vi "max clamp working in light.vi"(0 "Image In":T4, 1 "Clamp Settings (Max Clamp 1)":T1={"Angle Range (+/-)"=10.0, "Edge Polarity"={"Start"=0, "End"=0}} {"Edge Polarity"."Start" items=["Any", "Rising", "Falling"]; "Edge Polarity"."End" items=["Any", "Rising", "Falling"]}, 7 "error in":errorcluster) -> (20 "Image Out":T4, 21 "Clamp Results (Max Clamp 1)":T3, 22 "Clamp Points (Max Clamp 1)":T2, 24 "X Average":dbl, 27 "error out":errorcluster)   [LabVIEW 2016]
uses:
  <vilib>/vision/Image Controls.llb/IMAQ Image.ctl
  <vilib>/vision/Pattern Matching.llb/IMAQ Curve Parameters.ctl
  <vilib>/vision/NI_Vision_Development_Module.lvlib
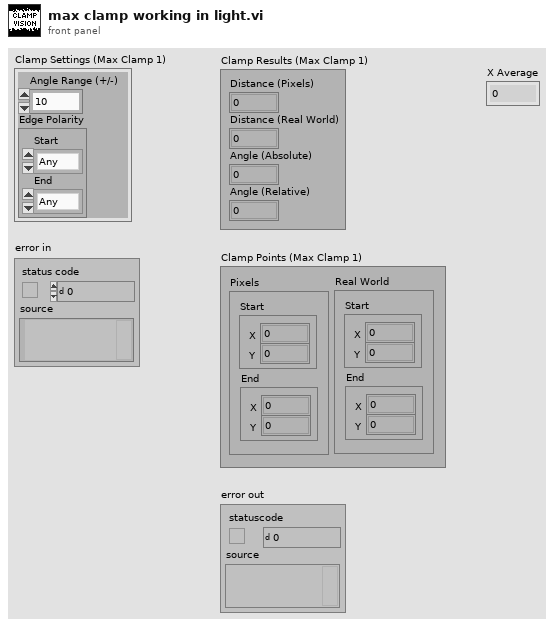
[diagram p1: front panel]
types:
  T1 = cluster{"Angle Range (+/-)":dbl, "Edge Polarity":cluster{"Start":u32, "End":u32}}
  T2 = cluster{"Pixels ":cluster{"Start":cluster{"X":dbl, "Y":dbl}, "End":cluster{"X":dbl, "Y":dbl}}, "Real World":cluster{"Start":cluster{"X":dbl, "Y":dbl}, "End":cluster{"X":dbl, "Y":dbl}}}
  T3 = cluster{"Distance (Pixels)":dbl, "Distance (Real World)":dbl, "Angle (Absolute)":dbl, "Angle (Relative)":dbl}
  T4 = typedef "IMAQ Image.ctl" = refnum<image>
  T5 = typedef "IMAQ Curve Parameters.ctl" = cluster{"Extraction Mode":u32, "Edge Threshold":i32, "Edge Filter Size":u32, "Min Length":i32, "Row Search Step Size":i32, "Col Search Step Size":i32, "Max Endpoint Gap":i32, "Closed":bool, "Subpixel":bool}
  T6 = cluster{"Show Search Area":bool, "Show Curves":bool, "Show Clamp Locations":bool, "Show Result":bool, "Search Area Color":u32, "Curves Color":u32, "Clamp Locations Color":u32, "Result Color":u32, "Overlay Group Name":string}
  T7 = cluster{"Global Rectangle":i32[], "Contours":cluster{"ID":enum32{"External", "Internal"}, "Type":u32, "Coordinates":i32[]}[]}
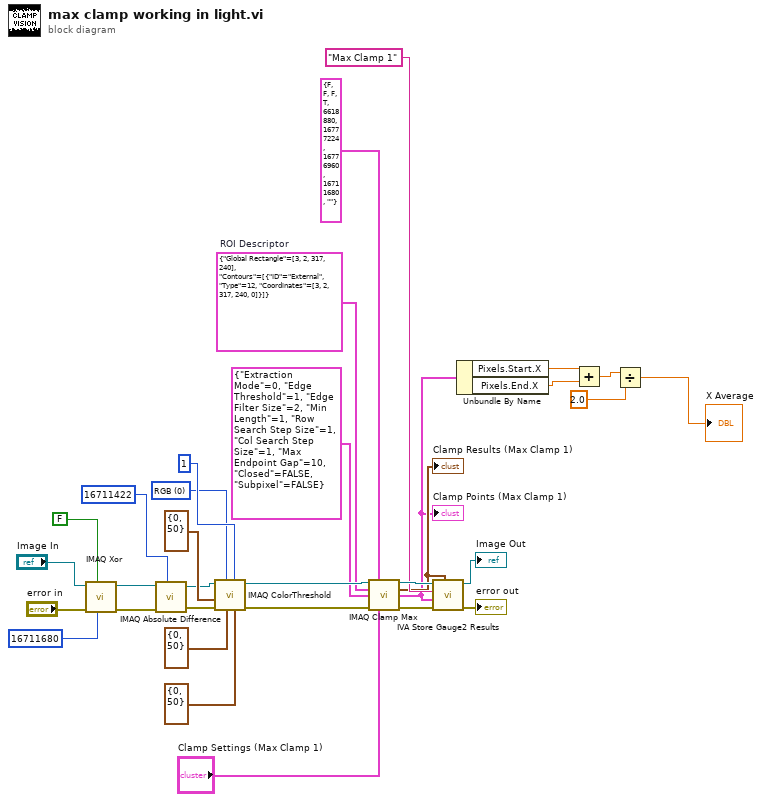
[diagram p0: block diagram]
diagram:
  w10 = T7 {"Global Rectangle"=[3, 2, 317, 240], "Contours"=[{"ID"=enum."External", "Type"=12, "Coordinates"=[3, 2, 317, 240, 0]}]}  # ROI Descriptor
  w24 = u16 0 items=["RGB", "HSL", "HSV", "HSI"] ("Color Mode")
  n1 = call "IMAQ Xor"("Constant"=16711680, "Xor/Xnor (Xor)"=FALSE, "error in (no error)"="error in", "Image Src A"="Image In") -> ("error out"=w27:errorcluster, "Image Dst Out"=w26:T4)  [unwired: 2 in, 4 out]
  n2 = call "IMAQ Absolute Difference"("Image Src A"=w26, "Constant"=16711422, "error in (no error)"=w27) -> ("Image Dst Out"=w20:T4, "error out"=w19:errorcluster)  [unwired: 2 in, 2 out]
  n3 = call "IMAQ ColorThreshold"("Blue or Luma or Val or Inten Range"=cluster{"Lower value":i32, "Upper value":i32} {"Lower value"=0, "Upper value"=50}, "Replace Value"=1, "Green or Sat Range"=cluster{"Lower value":i32, "Upper value":i32} {"Lower value"=0, "Upper value"=50}, "Color Mode"=w24, "error in (no error)"=w19, "Red or Hue Range"=cluster{"Lower value":i32, "Upper value":i32} {"Lower value"=0, "Upper value"=50}, "Image Src"=w20) -> ("error out"=w16:errorcluster, "Image Dst Out"=w17:T4)  [unwired: 1 in, 2 out]
  n4 = call "IMAQ Clamp Max"("Source Image"=w17, "Overlay Settings"=T6 {"Show Search Area"=FALSE, "Show Curves"=FALSE, "Show Clamp Locations"=FALSE, "Show Result"=TRUE, "Search Area Color"=6618880, "Curves Color"=16777224, "Clamp Locations Color"=16776960, "Result Color"=16711680, "Overlay Group Name"=""}, "ROI Descriptor"=w10, "Curve Extraction Settings"=T5 {"Extraction Mode"=0, "Edge Threshold"=1, "Edge Filter Size"=2, "Min Length"=1, "Row Search Step Size"=1, "Col Search Step Size"=1, "Max Endpoint Gap"=10, "Closed"=FALSE, "Subpixel"=FALSE}, "error in (no error)"=w16, "Clamp Settings"="Clamp Settings (Max Clamp 1)") -> ("Image Out"=w15:T4, "Clamp Results"=w7:T3, "Clamp Points"=w2:T2, "error out"=w18:errorcluster)  [unwired: 1 in, 5 out]
  "Clamp Results (Max Clamp 1)" <- w7
  "Clamp Points (Max Clamp 1)" <- w2
  n5 = call <vilib>:"IVA Store Gauge2 Results.vi"("Clamp Results"=w7, "error in (no error)"=w18, "Clamp Points"=w2, "Step Name"="Max Clamp 1", "Image in"=w15) -> ("error out"=→"error out":errorcluster, "Image Out"=→"Image Out":T4)  [unwired: 5 out]
  n6 = Unbundle By Name(w2) -> ("Pixels.Start.X"=w6:dbl, "Pixels.End.X"=w5:dbl)
  n7 = Add(x=w6, y=w5) -> (x+y=w4:dbl)
  n8 = Divide(x=w4, y=2.0) -> (x/y=→"X Average":dbl)
